vi "Acquire.vi"(6 "Acquisition":refnum<queue>, 8 "error in (no error)":errorcluster, 9 "Data Queue":refnum<queue>, 10 "Data Notifier":refnum<notifier>, 11 "Hardware Resources in":T1) -> (0 "error out":errorcluster, 3 "Hardware Resources out":T1)   [LabVIEW 2022 SP3, in "Acquisition.lvlib"]
doc: "Perform the acquisition. Replace the contents of this diagram with calls to acquisition hardware."
uses:
  Acquisition.lvlib
  Hardware Configuration.ctl
  Signal Type.ctl
  support/Message Queue/Message Cluster.ctl
  support/Message Queue/Message Queue.lvlib
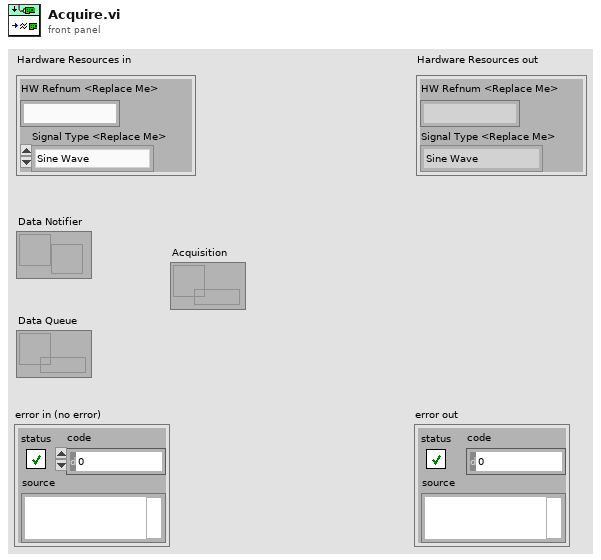
[diagram p1: front panel]
types:
  T1 = typedef "Acquisition.lvlib/Hardware Configuration.ctl" = cluster{"HW Refnum <Replace Me>":string, "Signal Type <Replace Me>":T2}
  T2 = typedef "Acquisition.lvlib/Signal Type.ctl" = enum16{"Sine Wave", "Square with Noise"}
  T3 = typedef "ClusterOut.ctl" = waveform(dbl)
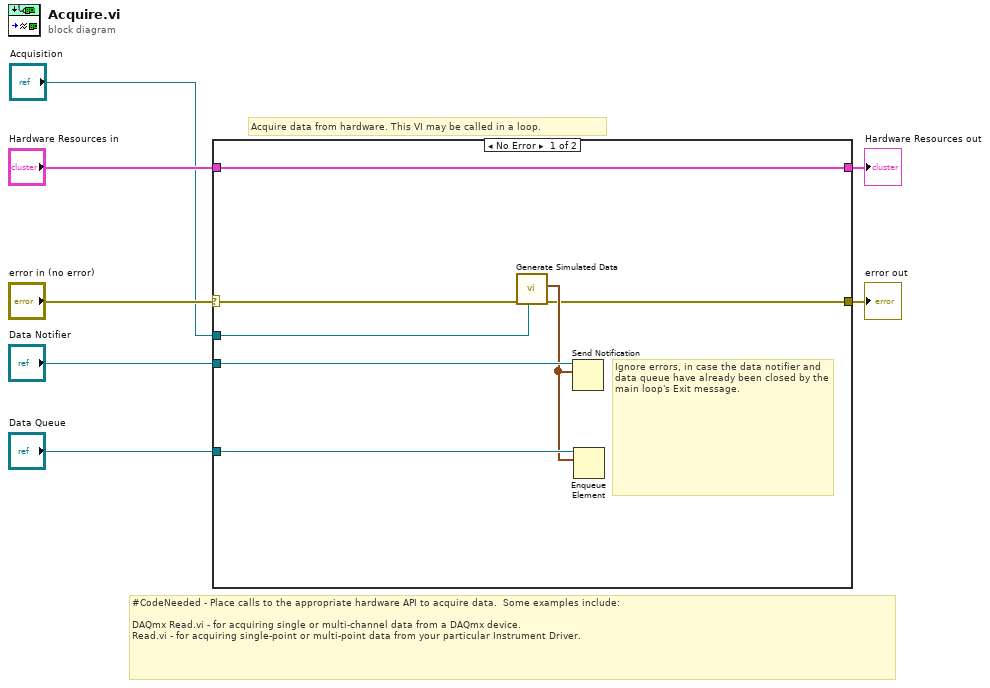
[diagram p0: block diagram]
diagram:
  # "Acquire data from hardware. This VI may be called in a loop."
  # "#CodeNeeded - Place calls to the appropriate hardware API to acquire data.  Some examples include:\n\nDAQmx Read.vi - for acquiring single or multi-channel data from a DAQmx device.\nRead.vi - for acquiring single-point or multi-point data from your particular Instrument Driver."
  n1 = case shown="No Error" "error in (no error)" {
    selector: "error in (no error)" -> [w14 w15]
    tunnel: [w10 w15] -> w6
    tunnel: "Hardware Resources in" -> [w8 w16]
    tunnel: [w8 w16] -> w4
    tunnel: "Data Notifier" -> [w13 _]
    tunnel: "Data Queue" -> [w12 _]
    tunnel: "Acquisition" -> [w9 _]
    frame No Error {
      # "Ignore errors, in case the data notifier and data queue have already been closed by the main loop's Exit message."
      n2 = call "Generate Simulated Data.vi"("Acquisition"=w9, "error in (no error)"=w14) -> ("error out"=w10:errorcluster, "Graph Data"=w11:T3[])  [unwired: 8 in]
      n3 = Send Notification(notification=w11, notifier=w13) -> ()  [unwired: 1 in, 2 out]
      n4 = Enqueue Element(queue=w12, element=w11) -> ()  [unwired: 2 in, 3 out]
    }
    frame Error {
    }
  }
  "Hardware Resources out" <- w4
  "error out" <- w6
